vi "Dashboard Main.vi"() -> ()   [LabVIEW 2018]
uses:
  <vilib>/Utility/miscctls.llb/LVRowAndColumnTypeDef.ctl
  <vilib>/event_ctls.llb/eventvkey.ctl
  <vilib>/Rock Robotics/Network Tables/NT Read Numeric Array.vi
  <vilib>/Rock Robotics/Network Tables/NT Write Boolean.vi
  <vilib>/Rock Robotics/Network Tables/NT Read Boolean.vi
  <vilib>/Rock Robotics/WPI/Dashboard/WPI_DashboardLogging Global.vi
panel:
  in  "Camera Settings Right":T1={"Frame Rate"=30, "Compression"=30, "Size"=1, "DB Camera Config"=FALSE} {"Frame Rate" scale=1.0..30.0; "Compression" scale=100.0..-1.0; "Size" items=["640x480", "320x240", "160x120"]}
  in  "Camera Name Right":string(combo)="No Camera Selection"
  out "Camera Perf":string
  in  "Camera Settings":T1={"Frame Rate"=30, "Compression"=30, "Size"=1, "DB Camera Config"=FALSE} {"Frame Rate" scale=1.0..30.0; "Compression" scale=100.0..-1.0; "Size" items=["640x480", "320x240", "160x120"]}
  in  "TCP":refnum<k5>
  in  "Rec Mode":enum32{"Stop", "Record", "Playback"}(radio)
  out "Robot IP":string
  out "Image Message":string="Timeout in Camera Communications"
  in  "Dashboard Tab":T2(tab)
  in  "Bypass":bool
  out "Actif?":bool
  out "Limit Droite":bool
  out "Limit Gauche":bool
  out "Position Pendule":dbl
  out "Arr D":bool
  out "Arr G":bool
  out "Av D":bool
  out "Photocells":bool
  in  "Select Auto":string(combo)="Select Autonomous ..."
  out "NT Connection":bool
  out "MotorChart R":cluster{"Numeric":dbl, "Numeric":dbl}(graph)
  out "MotorChart L":cluster{"Numeric":dbl, "Numeric":dbl}(graph)
  out "MotorSliders R":cluster{"MotorSlide1":dbl, "MotorSlide2":dbl} {"MotorSlide2" scale=-1.0..1.0 scale format="%#_2e"; "MotorSlide1" scale=-1.0..1.0 scale format="%#_2e"}
  out "MotorSliders L":cluster{"MotorSlide1":dbl, "MotorSlide2":dbl} {"MotorSlide2" scale=-1.0..1.0 scale format="%#_2e"; "MotorSlide1" scale=-1.0..1.0 scale format="%#_2e"}
  out "Gyro":dbl(knob) scale=0.0..360.0
  out "JS1 Z":dbl(slide) scale=-1.0..1.0 scale format="%#_2e"
  out "JS1 Graph":cluster{"X":dbl, "Y":dbl}[](graph)
  out "JS1 Buttons":T3
  out "JS2 Z":dbl(slide) scale=-1.0..1.0 scale format="%#_2e"
  out "JS2 Graph":cluster{"X":dbl, "Y":dbl}[](graph)
  out "JS2 Buttons":T3
  out "Mode":T4(ring)=enum."Auto Disabled"
  out "Right Camera Perf":cluster{"Bandwidth (Mbps)":dbl, "FPS":dbl}
  out "Camera Image Right":T5(plugin-control)
  in  "DB/String 9":string
  in  "DB/String 8":string
  in  "DB/String 7":string
  in  "DB/String 6":string
  in  "DB/String 5":string
  in  "DB/String 4":string
  in  "DB/String 3":string
  in  "DB/String 2":string
  in  "DB/String 1":string
  in  "DB/String 0":string
  in  "DB/Slider 0":dbl(slide) scale=0.0..5.0
  in  "DB/Slider 1":dbl(slide) scale=0.0..5.0
  in  "DB/Slider 2":dbl(slide) scale=0.0..5.0
  in  "DB/Slider 3":dbl(slide) scale=0.0..5.0
  out "DB/LED 3":bool
  out "DB/LED 2":bool
  out "DB/LED 1":bool
  out "DB/LED 0":bool
  in  "DB/Button 3":bool
  in  "DB/Button 2":bool
  in  "DB/Button 1":bool
  in  "DB/Button 0":bool caption="New Name"
  in  "Test Slider":dbl(slide) scale=0.0..100.0 scale format="%#_3g"
  in  "On/Off":bool caption="Solenoid"
  in  "Test Name":u16(ring) items=["Select the test to run..."]
  in  "Test Tree":string(tree)
  in  "Motor":cluster{"Value":dbl, "Enable":bool} {"Value" scale=-1.0..1.0 scale format="%#_3g"}
  out "Progress":T6 {"Test Progress" scale=0.0..100.0}
  in  "Rev/Fwd":cluster{"Forward":bool, "Reverse":bool}
  in  "Test Ring":u16(ring) items=["Monochrome", "Color"]
  out "Cmd Status":string
  in  "Execute Command":bool
  in  "Command Params":string[][](table)
  in  "Command Selection":i32(listbox)
  in  "CheckList":i32(listbox)
  out "Tree":string(tree)
  out "Camera Image":T5(plugin-control)
  out "Background":bool
  in  "Camera Name":string(combo)="No Camera Selection"
  # "HW"
  # "HW"
  # "Joysticks"
  # "Drive Motors"
  # "Front"
  # "Right"
  # "Left"
  # "Back"
  # "This tab is a great place for autonomous settings and robot-specific values.\nPlace controls and indicators inside this tab and match name to\nDashboard Variables on robot. You can also delete this comment."
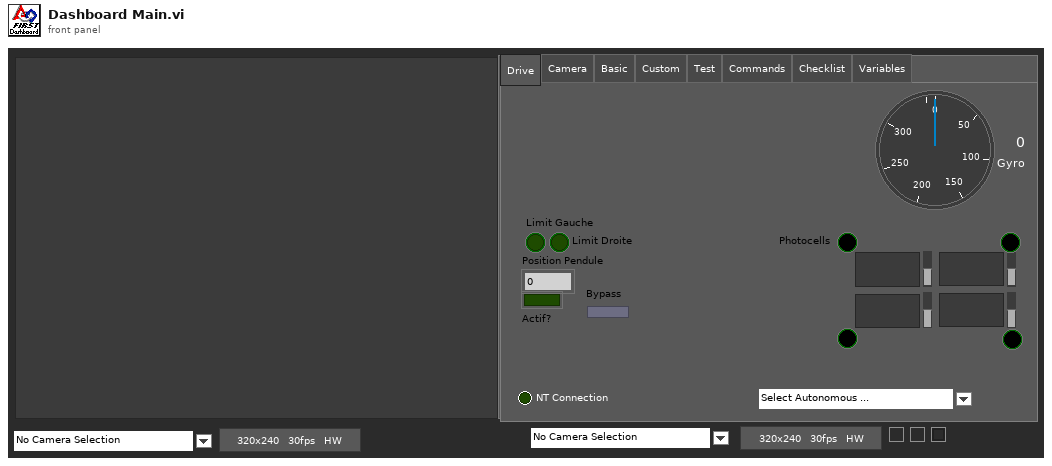
[diagram p1: front panel]
types:
  T1 = cluster{"Frame Rate":i32, "Compression":i32, "Size":u16, "DB Camera Config":bool}
  T2 = enum32{"Drive", "Camera", "Basic", "Custom", "Test", "Commands", "Checklist", "Variables"}
  T3 = cluster{bool, bool, bool, bool, bool, bool, bool, bool, bool, bool, bool, bool}
  T4 = enum8{"Tele-Op Disabled", "Tele-Op Enabled", "Auto Disabled", "Auto Enabled", "Test Disabled", "Test Enabled", "Disconnected", "No Code", "E-Stop"}
  T5 = typedef "IMAQ Image.ctl" = refnum<image>
  T6 = cluster{"Test Progress":u8, "Test Progress Text":string}
  T7 = cluster{"Save Path":path, "Interval (s)":dbl, "Keep":i32}
  T8 = typedef "Image Type" = u32
  T9 = cluster{"IDs":cluster{"RPC field ID":u16, "Unique ID":u16}, "String":string}
  T10 = cluster{"Error Strings":string, "Disable Counts":cluster{u16, u16}, "Rail Faults":cluster{u16, u16, u16}, "Robot IP":string, "DB Mode":u8, "Event Info":cluster{"Name":string, "Type":u8, "Number":u16, "Replay":u8}}
  T11 = cluster{"Storage":cluster{"Disk Free":u64, "RAM Block":u32, "RAM free":u32}, "CPU Utilization":cluster{"CPU % ISR":sgl, "CPU % Time Crit":sgl, "CPU % Timed Str":sgl, "CPU % High":sgl, "CPU % Above":sgl, "CPU % Normal":sgl, "CPU % Low":sgl}, "CAN":cluster{"% Bus Utilization":sgl, "Bus Off Cnt":u32, "TX_FIFO Full Cnt":u32, "Receive Error Cnt":u8, "Transmit Error Cnt":u8}, "HID":cluster{"HID Outputs":u32, "Rumble Low":u16, "Rumble High":u16}[]}
  T12 = cluster{"Status bits":cluster{"Test Mode":bool, "Autonomous":bool, "Enabled":bool, "Code Start":bool, "Brownout":bool, "Reserved 2":bool, "Reserved 3":bool, "E-Stop":bool}, "Code Trace":cluster{"Disabled":bool, "TeleOp":bool, "Auto":bool, "Test":bool}, "Controller Type":enum16{"unknown", "cRIO", "roboRio"}, "Code?":enum16{"unknown", "noCode", "code"}, "Battery V":dbl}
  T13 = cluster{"Control Bits":cluster{"TestMode":bool, "Autonomous":bool, "Enabled":bool, "FMS Present":bool, bool, bool, bool, "E-Stop":bool}, "Team Station ":u8, "Countdown":sgl, "Joystick Values":cluster{"Axes":dbl[], "Buttons":bool[], "POVs":i16[]}[]}
  T14 = cluster{"Axes":dbl[], "Buttons":bool[], "POVs":i16[]}[]
  T15 = cluster{"Axes":dbl[], "Buttons":bool[], "POVs":i16[]}
  T16 = cluster{"Buttons[0]":bool, "Buttons[1]":bool, "Buttons[2]":bool, "Buttons[3]":bool, "Buttons[4]":bool, "Buttons[5]":bool, "Buttons[6]":bool, "Buttons[7]":bool, "Buttons[8]":bool, "Buttons[9]":bool, "Buttons[10]":bool, "Buttons[11]":bool}
  T17 = cluster{"Camera Image":refnum<vi>, "Dashboard Tab":refnum<vi>, "Background":refnum<vi>, "Rec Mode":refnum<vi>, "Test Slider":refnum<vi>, "On/Off ":refnum<vi>, "Test Ring":refnum<vi>, "Rev/Fwd":refnum<vi>, "Test Name":refnum<vi>, "Motor":refnum<vi>, "Progress":refnum<vi>, "CheckList":refnum<vi>, "Tree":refnum<vi>, "Test Tree":refnum<vi>, "Command Params":refnum<vi>, "Command Selection":refnum<vi>, "Execute Command":refnum<vi>, "Cmd Status":refnum<vi>, "Camera Settings":refnum<vi>, "Camera Name":refnum<vi>, "Camera Perf":refnum<vi>, "Camera Settings Right":refnum<vi>, "Camera Name Right":refnum<vi>, "Camera Image Right":refnum<vi>}
  T18 = cluster{"Global Rectangle":i32[], "Contours":cluster{"Contour Type":u32, "ROI Type":u32, "Points":i32[]}[]}
  T19 = cluster{"Camera Name":string, string, "Saved DB Images Info":cluster{"Save Path":path, "Interval (s)":dbl, "Keep":i32}}
  T20 = cluster{"Camera Name Right":string, string, "Saved DB Images Info":cluster{"Save Path":path, "Interval (s)":dbl, "Keep":i32}}
  T21 = cluster{"Operation":enum16{"Update", "Clear"}, "Color Box":u32}[]
  T22 = typedef "eventvkey.ctl" = enum16{"ASCII", "Enter", "Return", "Shift", "Ctrl", "Alt", "Cmd", "Opt", "Caps", "NumLock", "Clear", "Break", "Up", "Down", "Left", "Right", "Insert", "Delete", "Home", "End", "PageUp", "PageDown", "Escape", "Help", "Pause", "ScrollLock", "F1", "F2", "F3", "F4", "F5", "F6", "F7", "F8", "F9", "F10", "F11", "F12", "F13", "F14", "F15", "F16", "F17", "F18", "F19", "F20", "F21", "F22", "F23", "F24", "Play", "VolumeUp", "VolumeDown", "Mute", "Two Byte Char"}
  T23 = cluster{"Image Size":bool, "Image Type":bool, "Pixel Value":bool, "ROI Information":bool, "Zoom Factor":bool}
  T24 = cluster{"Operation":enum16{"Update", "Clear"}, "Color Box":u32}
  T25 = typedef "LVRowAndColumnTypeDef.ctl" = cluster{"Row":i32, "Column":i32}
  T26 = cluster{"Shift":bool, "Ctrl":bool, "Alt":bool, "Cmd":bool, "Opt":bool}
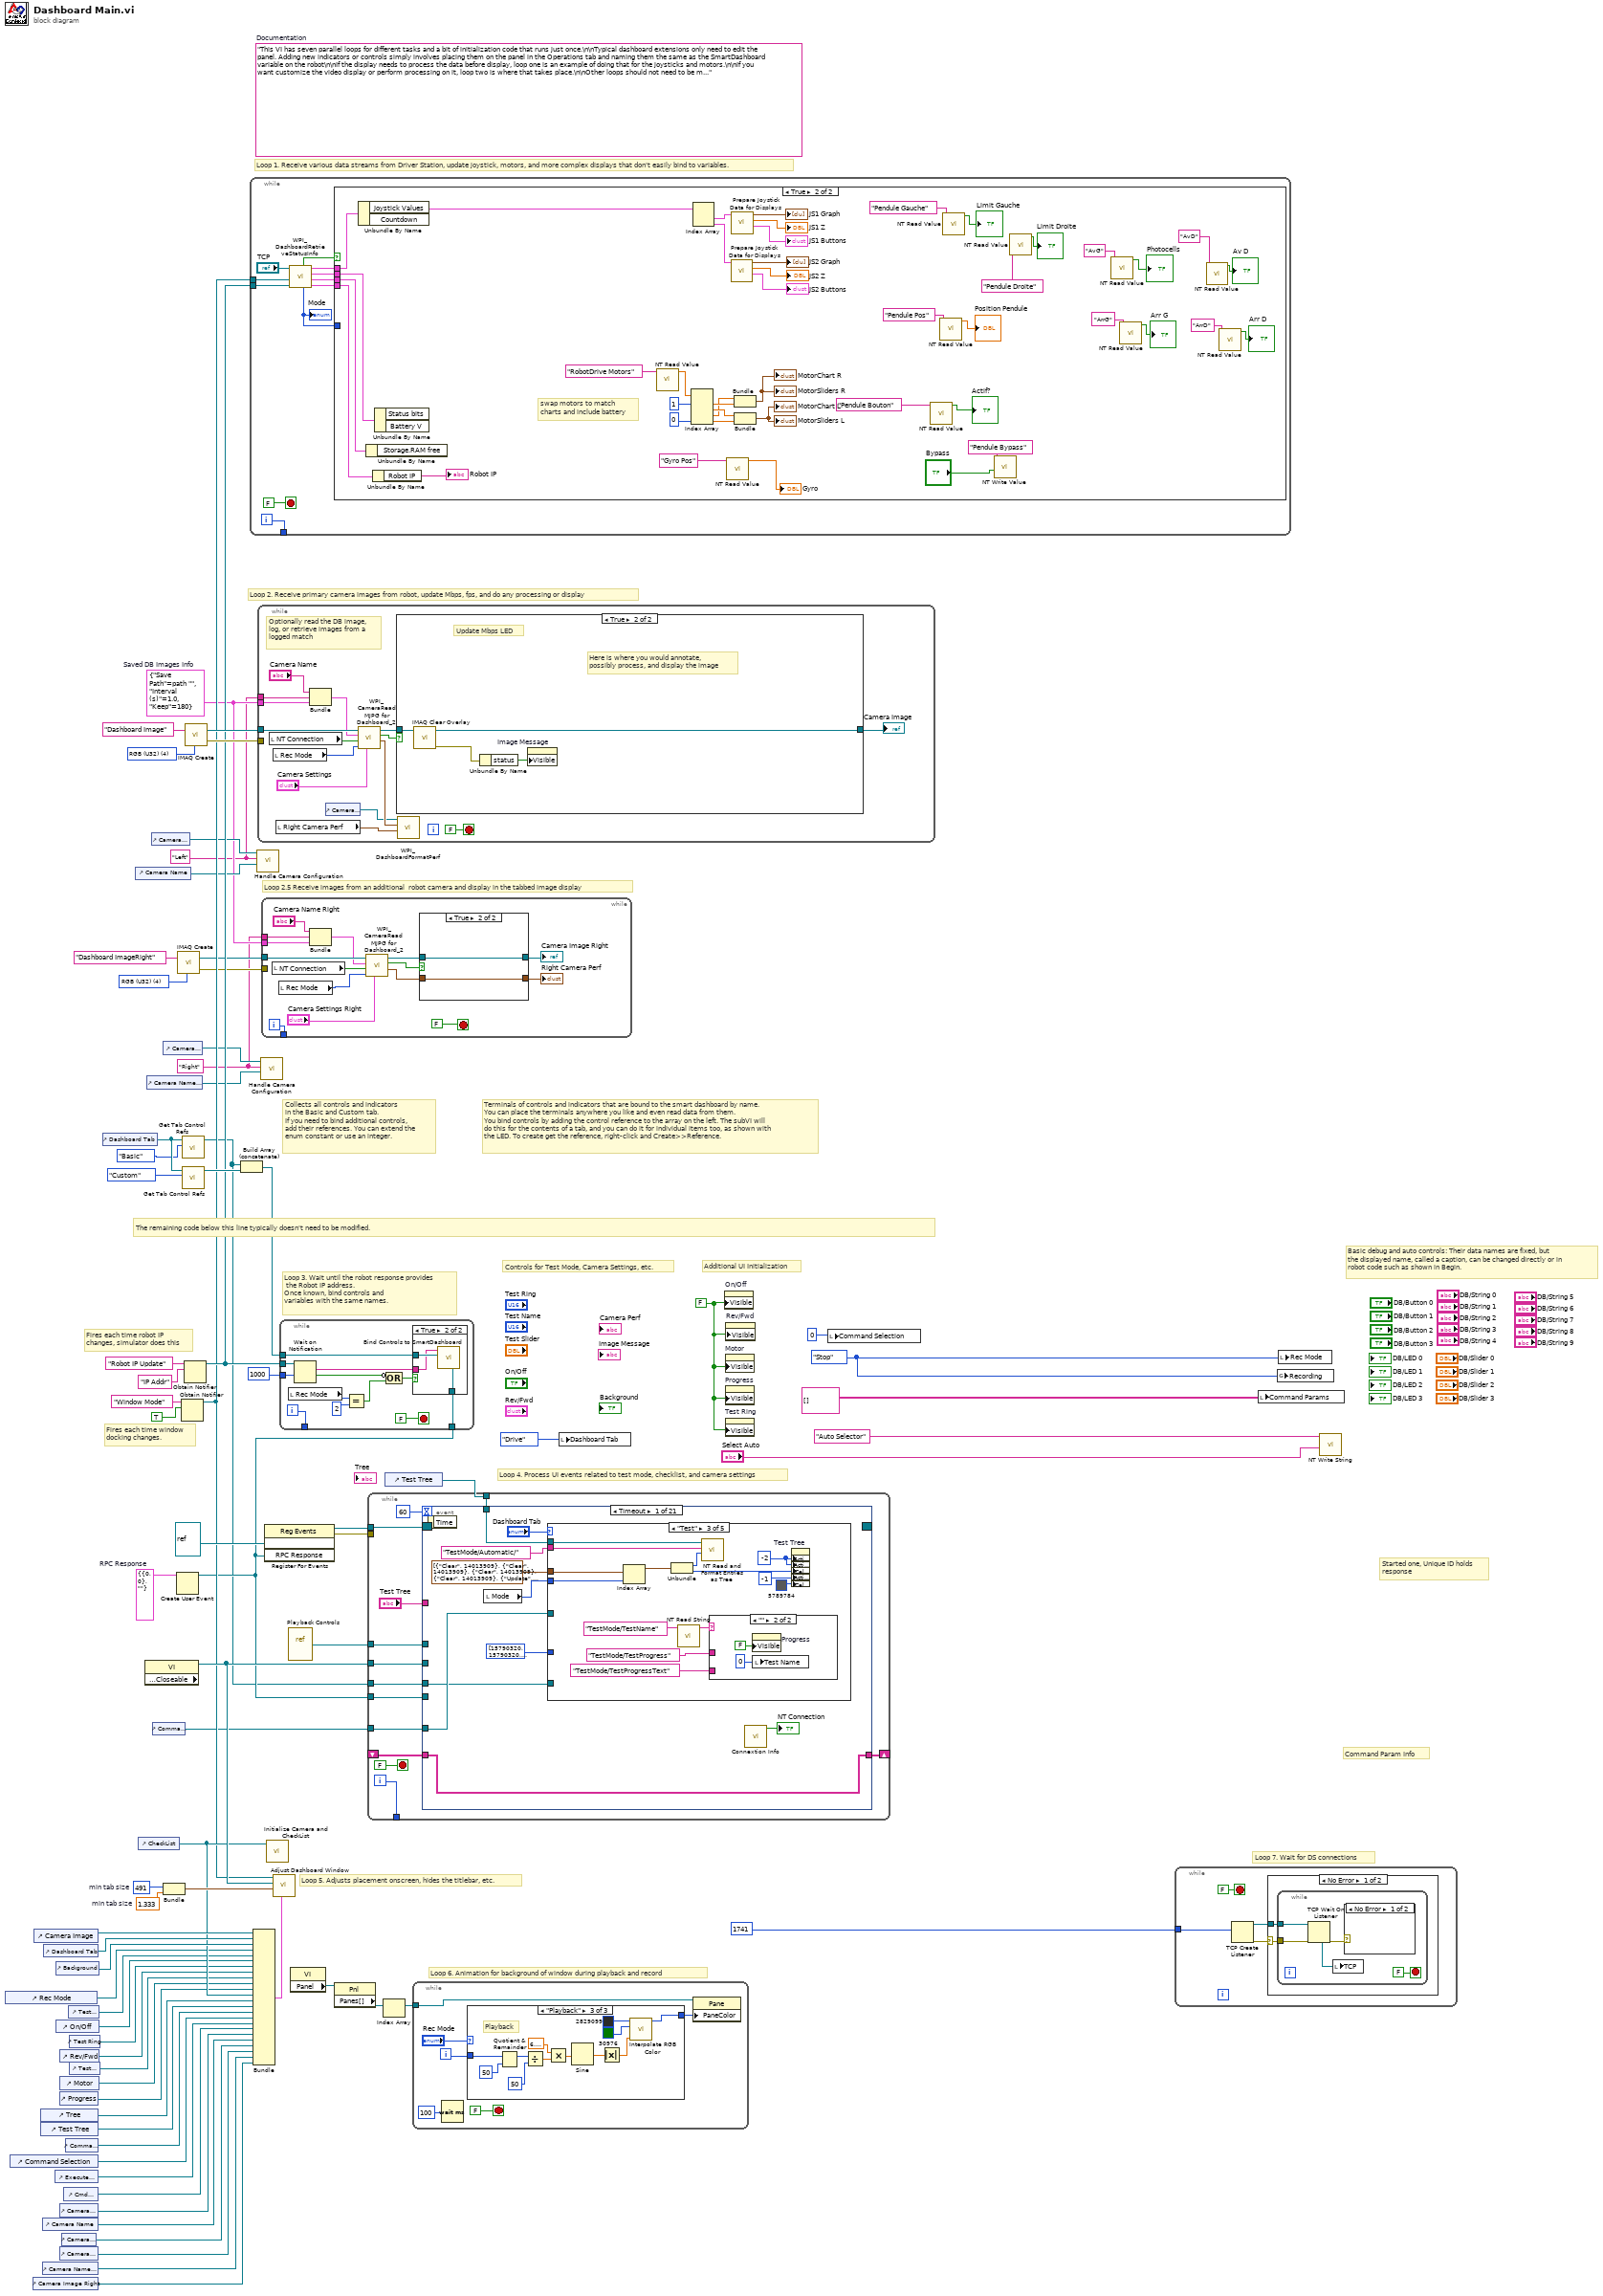
[diagram p0: block diagram]
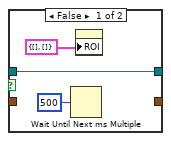
[diagram p2: hidden frame]
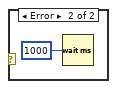
[diagram p3: hidden frame]
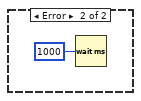
[diagram p4: hidden frame]
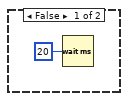
[diagram p5: hidden frame]
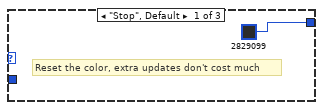
[diagram p6: hidden frame]
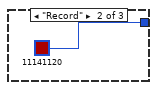
[diagram p7: hidden frame]
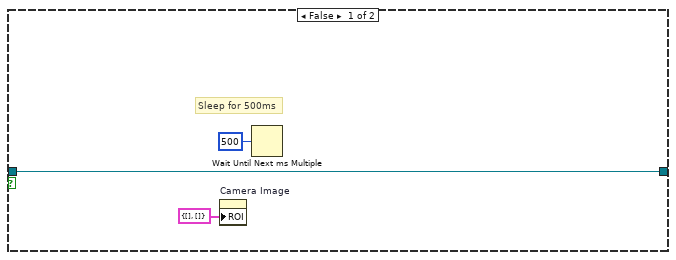
[diagram p9: hidden frame]
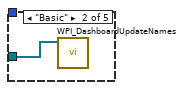
[diagram p11: hidden frame]
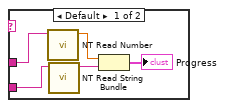
[diagram p12: hidden frame]
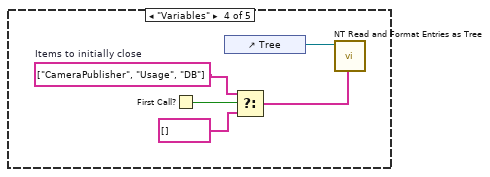
[diagram p13: hidden frame]
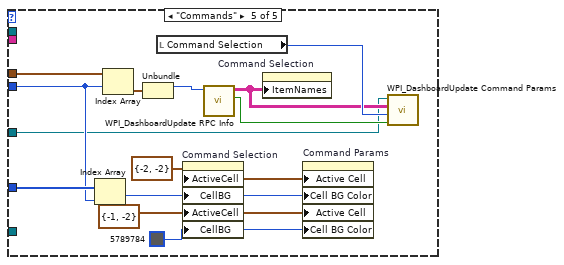
[diagram p14: hidden frame]
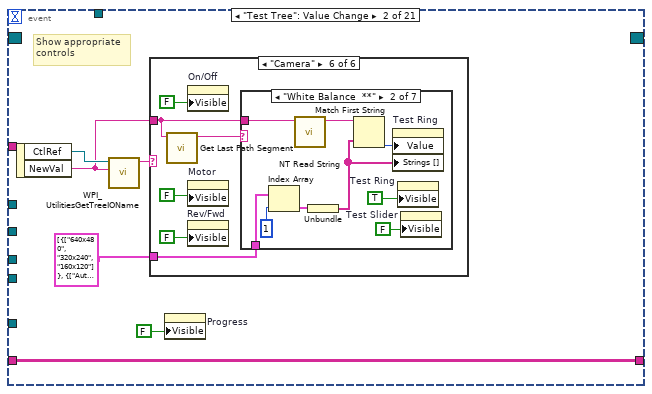
[diagram p15: hidden frame]
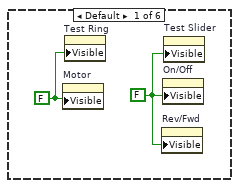
[diagram p16: hidden frame]
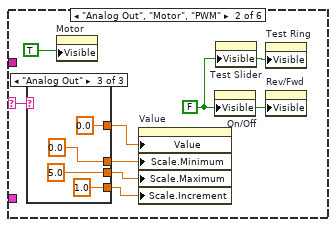
[diagram p17: hidden frame]
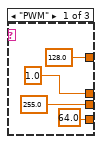
[diagram p18: hidden frame]
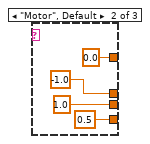
[diagram p19: hidden frame]
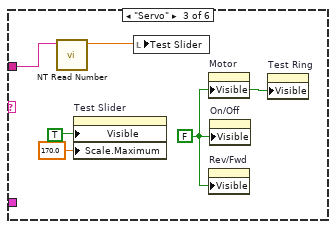
[diagram p20: hidden frame]
diagram:
  w3 = T7 {"Save Path"=path "", "Interval (s)"=1.0, "Keep"=180}  # Saved DB Images Info
  w2 = "Right"
  w1 = "Left"
  w13 = T8 4 items=["Grayscale (U8)", "Grayscale (I16)", "Grayscale (SGL)", "Complex (CSG)", "RGB (U32)", "HSL (U32)", "RGB (U64)"] ("Image Type")
  w29 = T9 {"IDs"={"RPC field ID"=0, "Unique ID"=0}, "String"=""}  # RPC Response
  w52 = 491  # min tab size
  w51 = 1.333  # min tab size
  w59 = enum32{"Stop", "Record", "Playback"}."Stop" ("Rec Mode")
  w36 = FALSE ("Visible")
  (unwired) "This VI has seven parallel loops for different tasks and a bit of initialization code that runs just once.\n\nTypical dashboard extensions only need to edit the panel. Adding new indicators or controls simply involves placing them on the panel in the Operations tab and naming them the same as the SmartDashboard variable on the robot\n\nIf the display needs to process the data before display, loop one is an example of doing that for the joysticks and motors.\n\nIf you want customize the video display or perform processing on it, loop two is where that takes place.\n\nOther loops should not need to be modified. They are pretty standard, and document the task they perform."  # Documentation
  w76 = T8 4 items=["Grayscale (U8)", "Grayscale (I16)", "Grayscale (SGL)", "Complex (CSG)", "RGB (U32)", "HSL (U32)", "RGB (U64)"] ("Image Type")
  # "Loop 2.5 Receive images from an additional  robot camera and display in the tabbed image display"
  # "Command Param Info"
  # "Started one, Unique ID holds\nresponse"
  # "Loop 7. Wait for DS connections"
  # "Basic debug and auto controls: Their data names are fixed, but\nthe displayed name, called a caption, can be changed directly or in\nrobot code such as shown in Begin."
  # "Controls for Test Mode, Camera Settings, etc."
  # "Additional UI Initialization"
  # "Loop 6. Animation for background of window during playback and record"
  # "Fires each time robot IP\nchanges, simulator does this"
  # "Fires each time window\ndocking changes."
  # "Collects all controls and indicators\nin the Basic and Custom tab.\nIf you need to bind additional controls,\nadd their references. You can extend the\nenum constant or use an integer."
  # "The remaining code below this line typically doesn't need to be modified."
  # "Loop 4. Process UI events related to test mode, checklist, and camera settings"
  # "Terminals of controls and indicators that are bound to the smart dashboard by name.\nYou can place the terminals anywhere you like and even read data from them.\nYou bind controls by adding the control reference to the array on the left. The subVI will\ndo this for the contents of a tab, and you can do it for individual items too, as shown with\nthe LED. To create get the reference, right-click and Create>>Reference."
  # "Loop 3. Wait until the robot response provides\n the Robot IP address.\nOnce known, bind controls and\nvariables with the same names."
  # "Loop 5. Adjusts placement onscreen, hides the titlebar, etc."
  # "Loop 1. Receive various data streams from Driver Station, update joystick, motors, and more complex displays that don't easily bind to variables."
  # "Loop 2. Receive primary camera images from robot, update Mbps, fps, and do any processing or display"
  n1 = control-ref of="Rec Mode"() -> (w42:refnum<vi>)
  n2 = control-ref of="Command Selection"() -> (w28:refnum<vi>)
  n3 = control-ref of="Camera Image Right"() -> (w6:refnum<vi>)
  n4 = control-ref of="Camera Image"() -> (w54:refnum<vi>)
  n5 = control-ref of="Tree"() -> (w46:refnum<vi>)
  n6 = control-ref of="Test Tree"() -> (w45:refnum<vi>)
  n7 = control-ref of="Camera Name"() -> (w19:refnum<vi>)
  n8 = control-ref of="Camera Name Right"() -> (w7:refnum<vi>)
  n9 = control-ref of="Dashboard Tab"() -> (w53:refnum<vi>)
  n10 = control-ref of="Execute Command"() -> (w30:refnum<vi>)
  n11 = control-ref of="Background"() -> (w49:refnum<vi>)
  n12 = control-ref of="On/Off"() -> (w40:refnum<vi>)
  n13 = control-ref of="Progress"() -> (w37:refnum<vi>)
  n14 = control-ref of="Camera Settings"() -> (w20:refnum<vi>)
  n15 = control-ref of="Camera Settings Right"() -> (w8:refnum<vi>)
  n16 = control-ref of="Rev/Fwd"() -> (w38:refnum<vi>)
  n17 = control-ref of="Motor"() -> (w43:refnum<vi>)
  n18 = control-ref of="Camera Perf"() -> (w18:refnum<vi>)
  n19 = control-ref of="Cmd Status"() -> (w24:refnum<vi>)
  n20 = control-ref of="Command Params"() -> (w31:refnum<vi>)
  n21 = control-ref of="Test Slider"() -> (w41:refnum<vi>)
  n22 = control-ref of="Test Ring"() -> (w39:refnum<vi>)
  n23 = control-ref of="Test Name"() -> (w44:refnum<vi>)
  n24 = control-ref of="Dashboard Tab"() -> (w57:refnum<vi>)
  n25 = control-ref of="Camera Name"() -> (w21:refnum<vi>)
  n26 = control-ref of="CheckList"() -> (w47:refnum<vi>)
  n27 = property class="VI" props=["Front Panel.Closeable"]() -> (reference out=w58:refnum<vi>)  [unwired: 2 in, 2 out]
  n28 = control-ref of="Camera Name Right"() -> (w9:refnum<vi>)
  n29 = control-ref of="Camera Settings"() -> (w22:refnum<vi>)
  n30 = control-ref of="Command Params"() -> (w23:refnum<vi>)
  n31 = control-ref of="Camera Settings Right"() -> (w10:refnum<vi>)
  n32 = Bundle("min tab size"=w52, "min tab size"=w51) -> (w50:cluster{"min tab size":i32, "min tab size":dbl})  [unwired: 1 in]
  n33 = Create User Event(user event datatype=w29) -> (user event=w25:refnum<user-event>)  [unwired: 1 in, 1 out]
  n34 = call "IMAQ Create"("Image Name"="Dashboard ImageRight", "Image Type"=w13) -> ("New Image"=w12:T5, "error out"=w11:errorcluster)  [unwired: 2 in, 1 out]
  n35 = Obtain Notifier(name (unnamed)="Window Mode", notification data type=TRUE) -> (notifier out=w34:refnum<notifier>)  [unwired: 2 in, 2 out]
  n36 = call <vilib>:"Get Tab Control Refs.vi"("Page Index"=T2."Basic" ("Dashboard Tab"), "TabControl in"=w57) -> ("ControlsOnPage"=w17:refnum<vi>[])  [unwired: 9 in]
  n37 = call <vilib>:"Get Tab Control Refs.vi"("Page Index"=T2."Custom" ("Dashboard Tab"), "TabControl in"=w57) -> ("ControlsOnPage"=w56:refnum<vi>[])  [unwired: 9 in]
  n38 = Obtain Notifier(name (unnamed)="Robot IP Update", notification data type="IP Addr" ("name (unnamed)")) -> (notifier out=w35:refnum<notifier>)  [unwired: 2 in, 2 out]
  n39 = call "IMAQ Create"("Image Name"="Dashboard Image", "Image Type"=w76) -> ("New Image"=w74:T5, "error out"=w73:errorcluster)  [unwired: 2 in, 1 out]
  n40 = Build Array (concatenate)(w17, w56) -> (w55:refnum<vi>[])
  n41 = while {
    tunnel: [w86] -> _
    tunnel: w35 -> [w80]
    tunnel: w34 -> [w77]
    i -> [w86]
    stop <- FALSE stop-if-true
    n42 = call <vilib>:"WPI_DashboardRetrieveStatusInfo.vi"("Binding Refnum"=w80, "Window Mode Notifier"=w77, "TCP Cnx"="TCP") -> ("Power and Errors"=w81:T10, "Robot Metrics"=w84:T11, "Status Info"=w85:T12, "Control Info"=w82:T13, "Robot Mode"=w79:T4, "Process?"=w83:bool)  [unwired: 3 in]
    "Mode" <- w79
    n43 = case shown="True" w83 {
      tunnel: w85 -> [_ w132]
      tunnel: w84 -> [_ w131]
      tunnel: w82 -> [_ w130]
      tunnel: w81 -> [_ w129]
      tunnel: w79 -> [_ _]
      frame False {
        n44 = Wait (ms)(milliseconds to wait=u32 20) -> ()  [unwired: 1 out]
      }
      frame True {
        # "swap motors to match\ncharts and include battery"
        n45 = Unbundle By Name(w130) -> ("Joystick Values"=w120:T14)  [unwired: 1 out]
        n46 = Unbundle By Name(w131) -> ()  [unwired: 1 out]
        n47 = Unbundle By Name(w129) -> ("Robot IP"=→"Robot IP":string)
        n48 = Unbundle By Name(w132) -> ()  [unwired: 2 out]
        n49 = call-poly <vilib>:"NT Read Value.vi"("Name"="RobotDrive Motors") -> ("Numeric Array"=w110:dbl[])  [unwired: 9 in, 1 out]
        n50 = Index Array(array=w110, index #1=1, index #4=0) -> (element #1=w124:dbl, element #2=w125:dbl, element #3=w123:dbl, element #4=w128:dbl)  [unwired: 2 in]
        n51 = Index Array(array=w120) -> (element #1=w119:T15, element #2=w115:T15)  [unwired: 2 in]
        n52 = call-poly <vilib>:"NT Read Value.vi"("Name"="Gyro Pos") -> ("Numeric"=→"Gyro":dbl)  [unwired: 9 in, 1 out]
        n53 = call "Prepare Joystick Data for Displays.vi"("Joystick Values"=w115) -> ("Buttons"=→"JS2 Buttons":T16, "Z Axis"=→"JS2 Z":dbl, "Cartesian Data"=→"JS2 Graph":cluster{"X axis":dbl, "X axis":dbl}[])  [unwired: 8 in]
        n54 = call "Prepare Joystick Data for Displays.vi"("Joystick Values"=w119) -> ("Buttons"=→"JS1 Buttons":T16, "Z Axis"=→"JS1 Z":dbl, "Cartesian Data"=→"JS1 Graph":cluster{"X axis":dbl, "X axis":dbl}[])  [unwired: 8 in]
        n55 = Bundle("Numeric"=w123, "Numeric"=w124) -> (→"MotorChart R" →"MotorSliders R":cluster{"Numeric":dbl, "Numeric":dbl})  [unwired: 1 in]
        n56 = Bundle("Numeric"=w125, "Numeric"=w128) -> (→"MotorChart L" →"MotorSliders L":cluster{"Numeric":dbl, "Numeric":dbl})  [unwired: 1 in]
        n57 = call-poly <vilib>:"NT Read Value.vi"("Name"="Pendule Bouton") -> ("Boolean"=→"Actif?":bool)  [unwired: 9 in, 1 out]
        n58 = call-poly <vilib>:"NT Read Value.vi"("Name"="Pendule Pos") -> ("Numeric"=→"Position Pendule":dbl)  [unwired: 9 in, 1 out]
        n59 = call-poly <vilib>:"NT Read Value.vi"("Name"="Pendule Gauche") -> ("Boolean"=→"Limit Gauche":bool)  [unwired: 9 in, 1 out]
        n60 = call-poly <vilib>:"NT Write Value.vi"("Boolean"="Bypass", "Name"="Pendule Bypass") -> ()  [unwired: 9 in, 1 out]
        n61 = call-poly <vilib>:"NT Read Value.vi"("Name"="Pendule Droite") -> ("Boolean"=→"Limit Droite":bool)  [unwired: 9 in, 1 out]
        n62 = call-poly <vilib>:"NT Read Value.vi"("Name"="AvG") -> ("Boolean"=→"Photocells":bool)  [unwired: 9 in, 1 out]
        n63 = call-poly <vilib>:"NT Read Value.vi"("Name"="ArrG") -> ("Boolean"=→"Arr G":bool)  [unwired: 9 in, 1 out]
        n64 = call-poly <vilib>:"NT Read Value.vi"("Name"="AvD") -> ("Boolean"=→"Av D":bool)  [unwired: 9 in, 1 out]
        n65 = call-poly <vilib>:"NT Read Value.vi"("Name"="ArrD") -> ("Boolean"=→"Arr D":bool)  [unwired: 9 in, 1 out]
      }
    }
  }
  n66 = Bundle("Camera Image"=w54, "Dashboard Tab"=w53, "Background"=w49, "Rec Mode"=w42, "Test Slider"=w41, "On/Off"=w40, "Test Ring"=w39, "Rev/Fwd"=w38, "Test Name"=w44, "Motor"=w43, "Progress"=w37, "CheckList"=w47, "Tree"=w46, "Test Tree"=w45, "Command Params"=w31, "Command Selection"=w28, "Execute Command"=w30, "Cmd Status"=w24, "Camera Settings"=w20, "Camera Name"=w19, "Camera Perf"=w18, "Camera Settings Right"=w8, "Camera Name Right"=w7, "Camera Image Right"=w6) -> (w48:T17)  [unwired: 1 in]
  n67 = call "Handle Camera Configuration.vi"("CameraNameRef"=w21, "Display Name"=w1, "ClusterRef"=w22) -> ()  [unwired: 9 in]
  n68 = while {
    tunnel: w74 -> [w146]
    tunnel: w73 -> [_]
    tunnel: w3 -> [w139]
    tunnel: w1 -> [w136]
    stop <- FALSE stop-if-true
    # "Optionally read the DB image,\nlog, or retrieve images from a\nlogged match"
    n69 = local read "NT Connection"() -> (w140:bool)
    n70 = local read "Rec Mode"() -> (w143:enum32{"Stop", "Record", "Playback"})
    n71 = local read "Right Camera Perf"() -> (w134:cluster{"Bandwidth (Mbps)":dbl, "FPS":dbl})
    n72 = Bundle("Camera Name"="Camera Name", w136, "Saved DB Images Info"=w139) -> (w138:T19)  [unwired: 1 in]
    n73 = control-ref of="Camera Perf"() -> (w133:refnum<vi>)
    n74 = call <vilib>:"WPI_CameraRead MJPG for Dashboard_2.vi"("Camera Settings"="Camera Settings", "Rec Mode"=w143, "NT Connection"=w140, "Capture Info"=w138, "Image in"=w146) -> ("perf info"=w135:cluster{"Bandwidth (Mbps)":dbl, "fps":dbl}, "Active"=w144:bool, "Image\\ out"=w145:T5)  [unwired: 4 in]
    n75 = case shown="True" w144 {
      tunnel: w145 -> [w149 w152]
      tunnel: [w149 w151] -> w141
      frame False {
        # "Sleep for 500ms"
        n76 = property on="Camera Image" class="ImageControl"("ROI"=T18 {"Global Rectangle"=[], "Contours"=[]}) -> ()  [unwired: 2 in, 2 out]
        n77 = Wait Until Next ms Multiple(millisecond multiple=u32 500) -> ()  [unwired: 1 out]
      }
      frame True {
        # "Here is where you would annotate,\npossibly process, and display the image"
        # "Update Mbps LED"
        n78 = call "IMAQ Clear Overlay"("Image"=w152) -> ("error out"=w153:errorcluster, "Image Out"=w151:T5)  [unwired: 2 in, 7 out]
        n79 = Unbundle By Name(w153) -> ("status"=w154:bool)
        n80 = property on="Image Message" class="Str"("Visible"=w154) -> ()  [unwired: 2 in, 2 out]
      }
    }
    "Camera Image" <- w141
    n81 = call <vilib>:"WPI_DashboardFormatPerf.vi"("Right Camera Perf"=w134, "Performance"=w135, "String in"=w133) -> ()  [unwired: 9 in]
  }
  n82 = call "Handle Camera Configuration.vi"("CameraNameRef"=w9, "Display Name"=w2, "ClusterRef"=w10) -> ()  [unwired: 9 in]
  n83 = while {
    tunnel: w12 -> [w169]
    tunnel: w11 -> [_]
    tunnel: [w164] -> _
    tunnel: w3 -> [w160]
    tunnel: w2 -> [w157]
    i -> [w164]
    stop <- FALSE stop-if-true
    n84 = local read "NT Connection"() -> (w161:bool)
    n85 = local read "Rec Mode"() -> (w168:enum32{"Stop", "Record", "Playback"})
    n86 = Bundle("Camera Name Right"="Camera Name Right", w157, "Saved DB Images Info"=w160) -> (w159:T20)  [unwired: 1 in]
    n87 = call <vilib>:"WPI_CameraRead MJPG for Dashboard_2.vi"("Camera Settings"="Camera Settings Right", "Rec Mode"=w168, "NT Connection"=w161, "Capture Info"=w159, "Image in"=w169) -> ("perf info"=w155:cluster{"Bandwidth (Mbps)":dbl, "fps":dbl}, "Active"=w163:bool, "Image\\ out"=w166:T5)  [unwired: 4 in]
    n88 = case shown="True" w163 {
      tunnel: w166 -> [w171 w174]
      tunnel: [w171 w174] -> w162
      tunnel: [_ w173] -> w156
      tunnel: w155 -> [_ w173]
      frame False {
        n89 = Wait Until Next ms Multiple(millisecond multiple=u32 500) -> ()  [unwired: 1 out]
        n90 = property on="Camera Image Right" class="ImageControl"("ROI"=T18 {"Global Rectangle"=[], "Contours"=[]}) -> ()  [unwired: 2 in, 2 out]
      }
      frame True {
      }
    }
    "Camera Image Right" <- w162
    "Right Camera Perf" <- w156
  }
  n91 = register-events(refnum<vi> refnum, w25) -> (reference out=w63:refnum<event-registration>, error out=w62:errorcluster)  [unwired: 2 in]
  n92 = call "Initialize Camera and CheckList.vi"("ListBox in"=w47) -> ()  [unwired: 11 in]
  n93 = call "Adjust Dashboard Window.vi"("Sizing Refnums"=w48, "Size Constraints"=w50, "VI"=w58, "WIn Mode"=w34) -> ()  [unwired: 8 in]
  n94 = while {
    tunnel: w55 -> [w186]
    tunnel: w35 -> [w184]
    tunnel: [w182] -> _
    tunnel: u32 1000 ("milliseconds to wait") -> [w181]
    tunnel: w25 -> [w175]
    i -> [w182]
    stop <- FALSE stop-if-true
    n95 = local read "Rec Mode"() -> (w177:enum32{"Stop", "Record", "Playback"})
    n96 = Wait on Notification(notifier=w184, timeout in ms (-1)=w181) -> (notification=w183:string, timed out?=w179:bool)  [unwired: 2 in, 2 out]
    n97 = Equal?(x=w177, y=u16 2 ("Rec Mode")) -> (x = y?=w178:bool)
    n98 = Compound Arithmetic op=OR(invert w179, w178) -> (w180:bool)
    n99 = case shown="True" w180 {
      tunnel: w186 -> [_ w189]
      tunnel: w183 -> [_ w188]
      tunnel: w175 -> [_ w187]
      frame False {
      }
      frame True {
        n100 = call <vilib>:"Bind Controls to SmartDashboard.vi"("RPC ref"=w187, "Bound Control Refs"=w189, "Server IP Address"=w188) -> ()  [unwired: 9 in]
      }
    }
  }
  n101 = vi-ref "Playback Controls.vi"() -> (w64:refnum<vi>)
  n102 = property class="VI"() -> ("Panel"=w66:refnum<vi>)  [unwired: 2 in, 2 out]
  n103 = property class="Pnl"(reference=w66) -> ("Panes[]"=w67:refnum<vi>[])  [unwired: 1 in, 2 out]
  n104 = Index Array(array=w67) -> (element=w65:refnum<vi>)  [unwired: 1 in]
  n105 = control-ref of="Test Tree"() -> (w68:refnum<vi>)
  n106 = while {
    tunnel: [w199] -> _
    tunnel: w68 -> [w198]
    tunnel: w64 -> [w197]
    tunnel: w63 -> [w196]
    tunnel: w62 -> [_]
    tunnel: w58 -> [w195]
    tunnel: w25 -> [w194]
    tunnel: w23 -> [w193]
    shift-right: [w192] -> _
    shift-left: _ -> [w191]
    tunnel: w17 -> [w190]
    i -> [w199]
    stop <- FALSE stop-if-true
    n107 = event shown="[0] Timeout" {
      selector: w196 -> [_ _ _ _ _ _ _ _ _ _ _ _ _ _ _ _ _ _ _ _ _]
      dyn-events: [_ _ _ _ _ _ _ _ _ _ _ _ _ _ _ _ w459 _ _ _ _] -> _
      timeout: u32 60 ("milliseconds to wait") -> [_ _ _ _ _ _ _ _ _ _ _ _ _ _ _ _ _ _ _ _ _]
      tunnel: w198 -> [w211 _ _ _ _ _ _ _ _ _ _ _ _ _ _ _ _ _ _ _ _]
      tunnel: "Test Tree" -> [_ _ _ _ _ _ _ _ _ _ _ w426 w434 w436 w440 w448 _ _ _ _ _]
      tunnel: w197 -> [_ _ _ _ _ _ _ _ _ _ _ _ _ _ _ _ w461 _ w479 _ _]
      tunnel: w195 -> [_ _ _ _ _ _ _ _ _ _ _ _ _ _ _ _ w457 _ _ _ _]
      tunnel: w194 -> [_ _ _ _ _ _ _ _ _ _ _ _ _ _ _ _ w455 _ _ _ _]
      tunnel: w193 -> [w206 _ _ _ _ _ w377 _ _ _ _ _ _ _ _ _ _ _ _ _ _]
      tunnel: [w205 w254 w356 w361 w370 w374 w375 w384 w394 w401 w413 w425 w432 w435 w439 w447 w454 w474 w476 w480 w493] -> w192
      tunnel: w191 -> [w205 w254 w356 w361 w370 w374 w375 _ _ w401 w413 w425 w432 w435 w439 w447 w454 w474 w476 w480 w493]
      tunnel: w190 -> [w203 _ _ _ _ _ _ _ _ _ _ _ _ _ _ _ _ _ _ _ _]
      event Timeout {
        n108 = event-data() -> ()  [unwired: 1 in, 1 out]
        n109 = local read "Mode"() -> (w208:T4)
        n110 = case shown="\"Test\"" "Dashboard Tab" {
          tunnel: w211 -> [_ _ w227 _ _]
          tunnel: "TestMode/Automatic/" ("Name Pattern") -> [_ _ w226 _ _]
          tunnel: T21 [{"Operation"=enum."Clear", "Color Box"=14013909}, {"Operation"=enum."Clear", "Color Box"=14013909}, {"Operation"=enum."Clear", "Color Box"=14013909}, {"Operation"=enum."Clear", "Color Box"=14013909}, {"Operation"=enum."Update", "Color Box"=14013909}, {"Operation"=enum."Update", "Color Box"=16777215}, {"Operation"=enum."Clear", "Color Box"=14013909}, {"Operation"=enum."Clear", "Color Box"=14013909}, {"Operation"=enum."Clear", "Color Box"=14013909}] -> [_ _ w219 _ w247]
          tunnel: w208 -> [_ _ w218 _ w246]
          tunnel: u32[] [15790320, 15790320, 15790320, 15790320, 16777215, 16777215, 15790320, 15790320, 15790320] -> [_ _ _ _ w252]
          tunnel: w206 -> [_ _ _ _ w240]
          tunnel: w203 -> [_ w213 _ _ _]
          frame "Custom", Default {
          }
          frame "Basic" {
            n111 = call <vilib>:"WPI_DashboardUpdateNames.vi"("Controls on Tab"=w213) -> ()  [unwired: 11 in]
          }
          frame "Test" {
            w225 = -2 ("Active Item:Row Number")
            n112 = Index Array(array=w219, index=w218) -> (element=w220:T24)
            n113 = Unbundle(w220) -> ("Operation"=w221:enum16{"Update", "Clear"}, "Color Box"=w222:u32)
            n114 = call <vilib>:"NT Read String.vi"("Name"="TestMode/TestName") -> ("String"=w216:string)  [unwired: 9 in, 1 out]
            n115 = call <vilib>:"NT Read and Format Entries as Tree.vi"("Operation"=w221, "Name Pattern"=w226, "Tree Refnum"=w227) -> ()  [unwired: 7 in, 2 out]
            n116 = case shown="\"\"" w216 {
              tunnel: "TestMode/TestProgress" ("Name") -> [w229 _]
              tunnel: "TestMode/TestProgressText" ("Name") -> [w228 _]
              frame Default {
                n117 = call <vilib>:"NT Read Number.vi"("Name"=w229) -> ("Numeric"=w230:dbl)  [unwired: 9 in, 1 out]
                n118 = call <vilib>:"NT Read String.vi"("Name"=w228) -> ("String"=w231:string)  [unwired: 9 in, 1 out]
                n119 = Bundle("Numeric"=w230, "String"=w231) -> (→"Progress":cluster{"Numeric":dbl, "String":string})  [unwired: 1 in]
              }
              frame "" {
                n120 = property on="Progress" class="Clust (strict)"("Visible"=FALSE) -> ()  [unwired: 2 in, 2 out]
                n121 = local write "Test Name"(u16 0) -> ()
              }
            }
            n122 = property on="Test Tree" class="Tree (strict)"("Active Item Row Number"=w225, "ActiveColNum"=w225, "CellBG"=w222, "Active Item Row Number"=-1 ("Active Item:Row Number"), "CellBG"=u32 5789784 ("Color Box")) -> ()  [unwired: 2 in, 2 out]
          }
          frame "Variables" {
            w237 = string[] ["CameraPublisher", "Usage", "DB"]  # Items to initially close
            n123 = First Call?() -> (First Call?: T/F=w238:bool)
            n124 = control-ref of="Tree"() -> (w239:refnum<vi>)
            n125 = Select(t=w237, s=w238, f=string[] []) -> (s? t:f=w235:string[])
            n126 = call <vilib>:"NT Read and Format Entries as Tree.vi"("Tags to  Close"=w235, "Tree Refnum"=w239) -> ()  [unwired: 8 in, 2 out]
          }
          frame "Commands" {
            w248 = u32 5789784 ("Color Box")
            w249 = T25 {"Row"=-1, "Column"=-2} ("Active Cell:Active Cell")
            w251 = T25 {"Row"=-2, "Column"=-2} ("Active Cell:Active Cell")
            n127 = Index Array(array=w252, index=w246) -> (element=w250:u32)
            n128 = Index Array(array=w247, index=w246) -> (element=w245:T24)
            n129 = Unbundle(w245) -> ("Operation"=w244:enum16{"Update", "Clear"})  [unwired: 1 out]
            n130 = local read "Command Selection"() -> (w243:i32)
            n131 = property on="Command Selection" class="MCListbox (strict)"("ActiveCell"=w251, "CellBG"=w250, "ActiveCell"=w249, "CellBG"=w248) -> ()  [unwired: 2 in, 2 out]
            n132 = call <vilib>:"WPI_DashboardUpdate RPC Info.vi"("Operation"=w244) -> ("update"=w242:bool, "commands"=w241:string[][])  [unwired: 9 in]
            n133 = property on="Command Selection" class="MCListbox (strict)"("ItemNames"=w241) -> ()  [unwired: 2 in, 2 out]
            n134 = property on="Command Params" class="Tbl (strict)"("Active Cell"=w251, "Cell BG Color"=w250, "Active Cell"=w249, "Cell BG Color"=w248) -> ()  [unwired: 2 in, 2 out]
            n135 = call <vilib>:"WPI_DashboardUpdate Command Params.vi"("Update"=w242, "NewVal"=w243, "Commands"=w241, "Param Tbl"=w240) -> ()  [unwired: 7 in, 1 out]
          }
        }
        n136 = call <vilib>:"Connextion Info.vi"() -> ("Connected"=→"NT Connection":bool)  [unwired: 10 in, 1 out]
      }
      event "Test Tree": Value Change {
        # "Show appropriate\ncontrols"
        n137 = event-data() -> ("CtlRef"=w257:refnum<vi>, "NewVal"=w255:string)  [unwired: 1 in]
        n138 = call <vilib>:"WPI_UtilitiesGetTreeIOName.vi"("NewVal"=w255, "TreeControl in"=w257) -> ("I/O Name"=w258:string)  [unwired: 9 in]
        n139 = case shown="\"Camera\"" w258 {
          selector: w258 -> [_ w265 _ w287 w296 _]
          tunnel: w255 -> [_ _ w284 w286 _ w303]
          tunnel: cluster{string[]}[] [{["640x480", "320x240", "160x120"]}, {["Auto", "Fixed indoor", "Fixed outdoor 1", "Fixed outdoor 2", "Fixed fluorescent 1", "Fixed fluorescent 2", "Hold current"]}, {["Auto", "Flicker-free 50 Hz", "Flicker-free 60 Hz", "Hold current"]}, {["None", "Prioritize frame rate", "Prioritize image quality"]}, {["Monochrome", "Color"]}] -> [_ _ _ _ _ w302]
          frame Default {
            w260 = FALSE ("Visible")
            w259 = FALSE ("Visible")
            n140 = property on="Motor" class="Clust (strict)"("Visible"=w259) -> ()  [unwired: 2 in, 2 out]
            n141 = property on="Test Ring" class="Ring (strict)"("Visible"=w259) -> ()  [unwired: 2 in, 2 out]
            n142 = property on="Rev/Fwd" class="Clust (strict)"("Visible"=w260) -> ()  [unwired: 2 in, 2 out]
            n143 = property on="On/Off" class="Bool (strict)"("Visible"=w260) -> ()  [unwired: 2 in, 2 out]
            n144 = property on="Test Slider" class="Slide (strict)"("Visible"=w260) -> ()  [unwired: 2 in, 2 out]
          }
          frame "Analog Out", "Motor", "PWM" {
            w266 = FALSE ("Visible")
            n145 = case shown="\"Analog Out\"" w265 {
              tunnel: [1.0 ("Value") -1.0 ("Value") 0.0 ("Value")] -> w264
              tunnel: [255.0 ("Value") 1.0 ("Value") 5.0 ("Value")] -> w263
              tunnel: [128.0 ("Value") 0.0 ("Value") 0.0 ("Value")] -> w262
              tunnel: [64.0 ("Value") 0.5 ("Value") 1.0 ("Value")] -> w261
              frame "PWM" {
              }
              frame "Motor", Default {
              }
              frame "Analog Out" {
              }
            }
            n146 = property on="Motor" class="Clust (strict)"("Visible"=TRUE) -> ()  [unwired: 2 in, 2 out]
            n147 = property on="Value" class="Slide (strict)"("Value"=w262, "Scale.Minimum"=w264, "Scale.Maximum"=w263, "Scale.Increment"=w261) -> ()  [unwired: 2 in, 2 out]
            n148 = property on="On/Off" class="Bool (strict)"("Visible"=w266) -> ()  [unwired: 2 in, 2 out]
            n149 = property on="Test Slider" class="Slide (strict)"("Visible"=w266) -> ()  [unwired: 2 in, 2 out]
            n150 = property on="Test Ring" class="Ring (strict)"("Visible"=w266) -> ()  [unwired: 2 in, 2 out]
            n151 = property on="Rev/Fwd" class="Clust (strict)"("Visible"=w266) -> ()  [unwired: 2 in, 2 out]
          }
          frame "Servo" {
            w282 = FALSE ("Visible")
            n152 = call <vilib>:"NT Read Number.vi"("Name"=w284) -> ("Numeric"=w283:dbl)  [unwired: 9 in, 1 out]
            n153 = property on="Test Slider" class="Slide (strict)"("Visible"=TRUE, "Scale.Maximum"=170.0 ("Scale.Range:Maximum")) -> ()  [unwired: 2 in, 2 out]
            n154 = local write "Test Slider"(w283) -> ()
            n155 = property on="Motor" class="Clust (strict)"("Visible"=w282) -> ()  [unwired: 2 in, 2 out]
            n156 = property on="Rev/Fwd" class="Clust (strict)"("Visible"=w282) -> ()  [unwired: 2 in, 2 out]
            n157 = property on="On/Off" class="Bool (strict)"("Visible"=w282) -> ()  [unwired: 2 in, 2 out]
            n158 = property on="Test Ring" class="Ring (strict)"("Visible"=w282) -> ()  [unwired: 2 in, 2 out]
          }
          frame "Relay", "Solenoid" {
            w285 = FALSE ("Visible")
            n159 = property on="Motor" class="Clust (strict)"("Visible"=w285) -> ()  [unwired: 2 in, 2 out]
            n160 = property on="Test Slider" class="Slide (strict)"("Visible"=w285) -> ()  [unwired: 2 in, 2 out]
            n161 = Search and Replace String(input string=w286, search string="/Value  **", replace string="/Direction") -> (result string=w292:string)  [unwired: 5 in, 3 out]
            n162 = property on="Test Ring" class="Ring (strict)"("Visible"=w285) -> ()  [unwired: 2 in, 2 out]
            n163 = call <vilib>:"NT Read String.vi"("Name"=w292) -> ("String"=w290:string)  [unwired: 9 in, 1 out]
            n164 = Equal?(x="Both directions", y=w290) -> (x = y?=w288:bool)
            n165 = Not(x=w288) -> (.not. x?=w289:bool)
            n166 = property on="Rev/Fwd" class="Clust (strict)"("Visible"=w288) -> ()  [unwired: 2 in, 2 out]
            n167 = property on="On/Off" class="Bool (strict)"("Visible"=w289, "Caption.Text"=w287) -> ()  [unwired: 2 in, 2 out]
          }
          frame "Compressor", "Digital Out" {
            w295 = FALSE ("Visible")
            # "Get direction and finish"
            n168 = property on="Motor" class="Clust (strict)"("Visible"=w295) -> ()  [unwired: 2 in, 2 out]
            n169 = property on="Test Slider" class="Slide (strict)"("Visible"=w295) -> ()  [unwired: 2 in, 2 out]
            n170 = property on="Test Ring" class="Ring (strict)"("Visible"=w295) -> ()  [unwired: 2 in, 2 out]
            n171 = property on="On/Off" class="Bool (strict)"("Visible"=TRUE, "Caption.Text"=w296) -> ()  [unwired: 2 in, 2 out]
            n172 = property on="Rev/Fwd" class="Clust (strict)"("Visible"=FALSE) -> ()  [unwired: 2 in, 2 out]
          }
          frame "Camera" {
            n173 = call <vilib>:"Get Last Path Segment.vi"("String in"=w303) -> ("String out"=w304:string)  [unwired: 10 in]
            n174 = property on="On/Off" class="Bool (strict)"("Visible"=FALSE) -> ()  [unwired: 2 in, 2 out]
            n175 = property on="Motor" class="Clust (strict)"("Visible"=FALSE) -> ()  [unwired: 2 in, 2 out]
            n176 = property on="Rev/Fwd" class="Clust (strict)"("Visible"=FALSE) -> ()  [unwired: 2 in, 2 out]
            n177 = case shown="\"White Balance  **\"" w304 {
              tunnel: w303 -> [w310 w319 w328 w337 w346 _ w352]
              tunnel: w302 -> [w308 w316 w325 w334 w343 _ _]
              frame "Size  **" {
                n178 = Index Array(array=w308) -> (element=w307:cluster{string[]})  [unwired: 1 in]
                n179 = call <vilib>:"NT Read String.vi"("Name"=w310) -> ("String"=w309:string)  [unwired: 9 in, 1 out]
                n180 = Unbundle(w307) -> (w305:string[])
                n181 = Match First String(2:w305, 3:w309) -> (0:w306:i32)  [unwired: 1 out]
                n182 = property on="Test Ring" class="Ring (strict)"("Value"=w306, "Strings []"=w305) -> ()  [unwired: 2 in, 2 out]
                n183 = property on="Test Ring" class="Ring (strict)"("Visible"=TRUE) -> ()  [unwired: 2 in, 2 out]
                n184 = property on="Test Slider" class="Slide (strict)"("Visible"=FALSE) -> ()  [unwired: 2 in, 2 out]
              }
              frame "White Balance  **" {
                n185 = Index Array(array=w316, index=1) -> (element=w317:cluster{string[]})
                n186 = call <vilib>:"NT Read String.vi"("Name"=w319) -> ("String"=w318:string)  [unwired: 9 in, 1 out]
                n187 = Unbundle(w317) -> (w314:string[])
                n188 = Match First String(2:w314, 3:w318) -> (0:w313:i32)  [unwired: 1 out]
                n189 = property on="Test Ring" class="Ring (strict)"("Value"=w313, "Strings []"=w314) -> ()  [unwired: 2 in, 2 out]
                n190 = property on="Test Ring" class="Ring (strict)"("Visible"=TRUE) -> ()  [unwired: 2 in, 2 out]
                n191 = property on="Test Slider" class="Slide (strict)"("Visible"=FALSE) -> ()  [unwired: 2 in, 2 out]
              }
              frame "Exposure  **" {
                n192 = Index Array(array=w325, index=2) -> (element=w326:cluster{string[]})
                n193 = call <vilib>:"NT Read String.vi"("Name"=w328) -> ("String"=w327:string)  [unwired: 9 in, 1 out]
                n194 = Unbundle(w326) -> (w322:string[])
                n195 = Match First String(2:w322, 3:w327) -> (0:w323:i32)  [unwired: 1 out]
                n196 = property on="Test Ring" class="Ring (strict)"("Value"=w323, "Strings []"=w322) -> ()  [unwired: 2 in, 2 out]
                n197 = property on="Test Ring" class="Ring (strict)"("Visible"=TRUE) -> ()  [unwired: 2 in, 2 out]
                n198 = property on="Test Slider" class="Slide (strict)"("Visible"=FALSE) -> ()  [unwired: 2 in, 2 out]
              }
              frame "Exposure Priority  **" {
                n199 = Index Array(array=w334, index=3) -> (element=w335:cluster{string[]})
                n200 = call <vilib>:"NT Read String.vi"("Name"=w337) -> ("String"=w336:string)  [unwired: 9 in, 1 out]
                n201 = Unbundle(w335) -> (w331:string[])
                n202 = Match First String(2:w331, 3:w336) -> (0:w332:i32)  [unwired: 1 out]
                n203 = property on="Test Ring" class="Ring (strict)"("Value"=w332, "Strings []"=w331) -> ()  [unwired: 2 in, 2 out]
                n204 = property on="Test Ring" class="Ring (strict)"("Visible"=TRUE) -> ()  [unwired: 2 in, 2 out]
                n205 = property on="Test Slider" class="Slide (strict)"("Visible"=FALSE) -> ()  [unwired: 2 in, 2 out]
              }
              frame "Color Enable  **" {
                n206 = Index Array(array=w343, index=4) -> (element=w344:cluster{string[]})
                n207 = call <vilib>:"NT Read String.vi"("Name"=w346) -> ("String"=w345:string)  [unwired: 9 in, 1 out]
                n208 = Unbundle(w344) -> (w340:string[])
                n209 = Match First String(2:w340, 3:w345) -> (0:w341:i32)  [unwired: 1 out]
                n210 = property on="Test Ring" class="Ring (strict)"("Value"=w341, "Strings []"=w340) -> ()  [unwired: 2 in, 2 out]
                n211 = property on="Test Ring" class="Ring (strict)"("Visible"=TRUE) -> ()  [unwired: 2 in, 2 out]
                n212 = property on="Test Slider" class="Slide (strict)"("Visible"=FALSE) -> ()  [unwired: 2 in, 2 out]
              }
              frame Default {
                n213 = property on="Test Ring" class="Ring (strict)"("Visible"=FALSE) -> ()  [unwired: 2 in, 2 out]
                n214 = property on="Test Slider" class="Slide (strict)"("Visible"=FALSE) -> ()  [unwired: 2 in, 2 out]
              }
              frame "Brightness  **", "Color Level  **", "Compression  **", "FPS  **", "Sharpness  **" {
                n215 = call <vilib>:"NT Read Number.vi"("Name"=w352) -> ("Numeric"=w351:dbl)  [unwired: 9 in, 1 out]
                n216 = local write "Test Slider"(w351) -> ()
                n217 = property on="Test Slider" class="Slide (strict)"("Visible"=TRUE, "Scale.Maximum"=100.0 ("Scale.Range:Maximum")) -> ()  [unwired: 2 in, 2 out]
                n218 = property on="Test Ring" class="Ring (strict)"("Visible"=FALSE) -> ()  [unwired: 2 in, 2 out]
              }
            }
          }
        }
        n219 = property on="Progress" class="Clust (strict)"("Visible"=FALSE) -> ()  [unwired: 2 in, 2 out]
      }
      event "Test Name": Mouse Enter {
        # "Populate the ring with the list of tests"
        n220 = event-data() -> ()  [unwired: 1 in, 1 out]
        n221 = call <vilib>:"NT Read String Array.vi"("Name"="TestMode/TestList") -> ("String Array"=w360:string[])  [unwired: 9 in, 1 out]
        n222 = Build Array (concatenate)("Select the test to run...", w360) -> (w359:string[])
        n223 = property on="Test Name" class="Ring (strict)"("Strings []"=w359) -> ()  [unwired: 2 in, 2 out]
      }
      event "Test Name": Value Change {
        w362 = FALSE ("Visible")
        # "Tell the robot the test name to run"
        n224 = event-data() -> ("NewVal"=w366:u16)  [unwired: 1 in]
        n225 = property on="Test Name" class="Ring (strict)"() -> ("Strings []"=w367:string[])  [unwired: 2 in, 2 out]
        n226 = local write "Progress"(T6 {"Test Progress"=0, "Test Progress Text"=""} ("Progress")) -> ()
        n227 = Index Array(array=w367, index=w366) -> (element=w365:string)
        n228 = call <vilib>:"NT Write String.vi"("String"=w365, "Name"="TestMode/TestName") -> ()  [unwired: 9 in, 1 out]
        n229 = property on="Progress" class="Clust (strict)"("Visible"=TRUE) -> ()  [unwired: 2 in, 2 out]
        n230 = property on="Motor" class="Clust (strict)"("Visible"=w362) -> ()  [unwired: 2 in, 2 out]
        n231 = property on="Test Slider" class="Slide (strict)"("Visible"=w362) -> ()  [unwired: 2 in, 2 out]
        n232 = property on="On/Off" class="Bool (strict)"("Visible"=w362) -> ()  [unwired: 2 in, 2 out]
        n233 = property on="Rev/Fwd" class="Clust (strict)"("Visible"=w362) -> ()  [unwired: 2 in, 2 out]
        n234 = property on="Test Ring" class="Ring (strict)"("Visible"=w362) -> ()  [unwired: 2 in, 2 out]
      }
      event "Select Auto": Mouse Enter {
        # "Populate the combo box with the list of autonomous options"
        n235 = event-data() -> ()  [unwired: 1 in, 1 out]
        n236 = call <vilib>:"NT Read String Array.vi"("Name"="Auto List") -> ("String Array"=w369:string[])  [unwired: 9 in, 1 out]
        n237 = property on="Select Auto" class="CmbBox"("Strings[]"=w369) -> ()  [unwired: 2 in, 2 out]
      }
      event "Select Auto": Value Change {
        # "User modified the Auto Selection. Write to NT variable so robot knows."
        n238 = event-data() -> ("NewVal"=w372:string)  [unwired: 1 in]
        n239 = call <vilib>:"NT Write String.vi"("String"=w372, "Name"="Auto Selector") -> ()  [unwired: 9 in, 1 out]
      }
      event "Command Selection": Value Change {
        # "Get the params and show in table"
        n240 = event-data() -> ("NewVal"=w378:i32)  [unwired: 1 in]
        n241 = property on="Command Selection" class="MCListbox (strict)"() -> ("ItemNames"=w376:string[][])  [unwired: 2 in, 2 out]
        n242 = call <vilib>:"WPI_DashboardUpdate Command Params.vi"("NewVal"=w378, "Commands"=w376, "Param Tbl"=w377) -> ()  [unwired: 8 in, 1 out]
      }
      event "Execute Command": Value Change {
        # "Started one, Unique ID holds\nresponse"
        n243 = event-data() -> ()  [unwired: 1 in, 1 out]
        n244 = property on="Command Selection" class="MCListbox (strict)"() -> ("ItemNames"=w389:string[][])  [unwired: 2 in, 2 out]
        n245 = Index Array(array=w389, index (row)="Command Selection", index (col)=0) -> (element=w387:string)
        n246 = call <vilib>:"Invoke Commands.vi"("Command Params"="Command Params", "Function Name"=w387) -> ("Params"=w383:u8, "Started"=w382:bool)  [unwired: 7 in, 1 out]
        n247 = Array Subset(array="Command Params", length (row)=w383) -> (w384:string[][])  [unwired: 3 in]
        n248 = Select(t="Executing" ("Cmd Status"), s=w382, f="" ("Cmd Status")) -> (s? t:f=→"Cmd Status":string)
      }
      event "Command Selection": Double Click {
        n249 = event-data() -> ("Row"=w397:i32)  [unwired: 1 in]
        n250 = property on="Command Selection" class="MCListbox (strict)"() -> ("ItemNames"=w400:string[][])  [unwired: 2 in, 2 out]
        n251 = local read "Command Params"() -> (w396:string[][])
        n252 = Index Array(array=w400, index (row)=w397, index (col)=0) -> (element=w398:string)
        n253 = call <vilib>:"Invoke Commands.vi"("Command Params"=w396, "Function Name"=w398) -> ("Params"=w395:u8, "Started"=w390:bool)  [unwired: 7 in, 1 out]
        n254 = Array Subset(array=w396, length (row)=w395) -> (w394:string[][])  [unwired: 3 in]
        n255 = Select(t="Executing" ("Cmd Status"), s=w390, f="" ("Cmd Status")) -> (s? t:f=w391:string)
        n256 = local write "Cmd Status"(w391) -> ()
      }
      event "CheckList": Double Click {
        # "Shift clears all"
        # "Update symbols on the listbox"
        n257 = event-data() -> ("PlatMods.Shift"=w402:bool, "Row"=w404:i32)  [unwired: 1 in]
        n258 = case shown="True" w402 {
          tunnel: w404 -> [w408 _]
          tunnel: 1 -> [w407 _]
          frame False {
            n259 = property on="CheckList" class="LstBox (strict)"() -> ("Item Symbols"=w406:i32[])  [unwired: 2 in, 2 out]
            n260 = Replace Array Subset(array=w406, new element=w407, index=w408) -> (w405:i32[])
            n261 = property on="CheckList" class="LstBox (strict)"("Item Symbols"=w405) -> ()  [unwired: 2 in, 2 out]
          }
          frame True {
            w409 = 0 ("Top Row")
            n262 = property on="CheckList" class="LstBox (strict)"() -> ("Number of Rows"=w411:u32)  [unwired: 2 in, 2 out]
            n263 = Initialize Array(0, w411) -> (w410:i32[])
            n264 = property on="CheckList" class="LstBox (strict)"("Top Row"=w409, "Value"=w409, "Item Symbols"=w410) -> ()  [unwired: 2 in, 2 out]
          }
        }
      }
      event "CheckList": Key Down {
        # "Update symbols on the listbox\nLeft and right keys check and uncheck"
        n265 = event-data() -> ("VKey"=w415:T22)  [unwired: 1 in]
        n266 = case shown="\"Left\", \"Right\"" w415 {
          selector: w415 -> [w420 _]
          tunnel: eventvkey."Left" ("VKey") -> [w418 _]
          frame "Left", "Right" {
            n267 = Equal?(x=w418, y=w420) -> (x = y?=w419:bool)
            n268 = Select(t=0, s=w419, f=1) -> (s? t:f=w421:i32)
            n269 = property on="CheckList" class="LstBox (strict)"() -> ("Item Symbols"=w424:i32[])  [unwired: 2 in, 2 out]
            n270 = Replace Array Subset(array=w424, new element=w421, index="CheckList") -> (w423:i32[])
            n271 = property on="CheckList" class="LstBox (strict)"("Item Symbols"=w423) -> ()  [unwired: 2 in, 2 out]
          }
          frame Default {
          }
        }
      }
      event "Motor.Enable": Value Change {
        # "When the test mode otor enable helper is set, update that\ntree row item's value"
        n272 = event-data() -> ("NewVal"=w430:bool)  [unwired: 1 in]
        n273 = Unbundle("Motor") -> ("Value"=w429:dbl)  [unwired: 1 out]
        n274 = Select(t=w429, s=w430, f=0.0) -> (s? t:f=w427:dbl)
        n275 = call <vilib>:"NT Write Number.vi"("Numeric"=w427, "Name"=w426) -> ()  [unwired: 9 in, 1 out]
      }
      event "Test Slider": Value Change {
        # "When the test mode slider helper is set, update that\ntree row item's value"
        n276 = event-data() -> ("NewVal"=w433:dbl)  [unwired: 1 in]
        n277 = call <vilib>:"NT Write Number.vi"("Numeric"=w433, "Name"=w434) -> ()  [unwired: 9 in, 1 out]
      }
      event "On/Off": Value Change {
        # "When the test mode on/off helper value is set, update that\ntree row item's value"
        n278 = event-data() -> ("NewVal"=w438:bool)  [unwired: 1 in]
        n279 = Boolean To (0,1)(Boolean=w438) -> (0, 1=w437:i16)
        n280 = call <vilib>:"NT Write Number.vi"("Numeric"=w437, "Name"=w436) -> ()  [unwired: 9 in, 1 out]
      }
      event "Rev/Fwd": Value Change {
        # "When the test mode helper value for relays is set, update that\ntree row item's value"
        n281 = event-data() -> ("NewVal.Forward"=w446:bool, "NewVal.Reverse"=w445:bool)  [unwired: 1 in]
        n282 = Boolean To (0,1)(Boolean=w446) -> (0, 1=w442:i16)
        n283 = Boolean To (0,1)(Boolean=w445) -> (0, 1=w444:i16)
        n284 = Negate(x=w444) -> (-x=w443:i16)
        n285 = Add(x=w442, y=w443) -> (x+y=w441:i16)
        n286 = call <vilib>:"NT Write Number.vi"("Numeric"=w441, "Name"=w440) -> ()  [unwired: 9 in, 1 out]
      }
      event "Test Ring": Value Change {
        # "When a test mode helper value is selected from the ring,\nset the tree item's variable to the string value"
        n287 = event-data() -> ("NewVal"=w450:u16)  [unwired: 1 in]
        n288 = property on="Test Ring" class="Ring (strict)"() -> ("Strings []"=w451:string[])  [unwired: 2 in, 2 out]
        n289 = Index Array(array=w451, index=w450) -> (element=w449:string)
        n290 = call <vilib>:"NT Write String.vi"("String"=w449, "Name"=w448) -> ()  [unwired: 9 in, 1 out]
      }
      event "Rec Mode": Value Change {
        # "Update globals for recording mode and path to read log from.\nClear when logging and let NetworkTables set path for vision to\nuse."
        n291 = event-data() -> ("NewVal"=w462:enum32{"Stop", "Record", "Playback"})  [unwired: 1 in]
        n292 = global write "WPI_DashboardLogging Global.vi" "Logging Filename"(path "") -> ()
        n293 = global write "WPI_DashboardLogging Global.vi" "Recording"(w462) -> ()
        n294 = case shown="\"Playback\"" w462 {
          tunnel: w461 -> [_ w464 w473]
          tunnel: [_ _ w472] -> w459
          tunnel: [_ _ w471] -> _
          tunnel: w457 -> [_ _ w469]
          tunnel: cluster{i32, i32} {-250, 170} -> [_ _ w468]
          tunnel: [_ _ T23 {"Image Size"=TRUE, "Image Type"=TRUE, "Pixel Value"=TRUE, "ROI Information"=TRUE, "Zoom Factor"=FALSE} ("Image Information Shown:All Elements")] -> w452
          tunnel: [_ _ TRUE ("Zoom Factor")] -> w453
          tunnel: w455 -> [_ _ w465]
          frame Default {
          }
          frame "Stop", "Record" {
            # "Place Window too"
            n295 = invoke class="VI" method="FP.Close"(reference=w464) -> (reference out=w463:refnum<vi>)  [unwired: 2 in, 2 out]
            n296 = invoke class="VI" method="Abort VI"(reference=w463) -> ()  [unwired: 2 in, 3 out]
          }
          frame "Playback" {
            n297 = call "Open Playback Panel.vi"("Offset"=w468, "DB VI Ref"=w469, "Playback in"=w473) -> ("Playback out"=w470:refnum<vi>)  [unwired: 8 in]
            n298 = register-events(w470, w465) -> (reference out=w472:refnum<event-registration>, error out=w471:errorcluster)  [unwired: 2 in]
          }
        }
        n299 = property on="Camera Image Right" class="ImageControl"("Image Information Shown"=w452, "Image Information Visible"=w453) -> ()  [unwired: 2 in, 2 out]
        n300 = property on="Camera Image" class="ImageControl"("Image Information Shown"=w452, "Image Information Visible"=w453) -> ()  [unwired: 2 in, 2 out]
        n301 = call <vilib>:"WPI_DashboardNT Log FieldName Cache.vi"("Operation"=enum16{"Lookup/Add", "Index", "Clear"}."Clear") -> ()  [unwired: 8 in, 3 out]
      }
      event Panel Close {
        w475 = enum32{"Stop", "Record", "Playback"}."Stop" ("Rec Mode")
        # "Playback window has been closed, abort"
        n302 = event-data() -> ()  [unwired: 1 in, 4 out]
        n303 = local write "Rec Mode"(w475) -> ()
        n304 = global write "WPI_DashboardLogging Global.vi" "Recording"(w475) -> ()
      }
      event Panel Close {
        # "Abort playback window and ourself"
        n305 = event-data() -> ()  [unwired: 1 in, 4 out]
        n306 = invoke class="VI" method="FP.Close"(reference=w479) -> (reference out=w478:refnum<vi>)  [unwired: 2 in, 2 out]
        n307 = invoke class="VI" method="Abort VI"(reference=w478) -> (error out=w477:errorcluster)  [unwired: 2 in, 2 out]
        n308 = invoke class="VI" method="Abort VI"(error in=w477) -> ()  [unwired: 2 in, 3 out]
      }
      event User Event {
        n309 = event-data() -> ("IDs"=w486:cluster{"RPC field ID":u16, "Unique ID":u16}, "String"=w485:string)  [unwired: 1 in]
        n310 = Bundle("IDs"=w486, "String"=w485) -> (w484:T9)  [unwired: 1 in]
        n311 = call <vilib>:"Retrieve RPC Response.vi"("RPC Response"=w484) -> ("Output"=w482:string[][])  [unwired: 10 in]
        n312 = Build Array (concatenate)(w480, w482) -> (w481:string[][])
        n313 = local write "Command Params"(w481) -> ()
        n314 = local write "Cmd Status"("" ("Cmd Status")) -> ()
      }
      event "Tree": Double Click {
        n315 = event-data() -> ("PlatMods"=w492:T26, "Tag"=w489:string)  [unwired: 1 in]
        n316 = Unbundle(w492) -> ("Shift"=w491:bool)  [unwired: 4 out]
        n317 = String Subset(string=w489, length (rest)=1 ("length (rest)")) -> (substring=w488:string)  [unwired: 1 in]
        n318 = Not(x=w491) -> (.not. x?=w490:bool)
        n319 = case shown="\"/\"" w488 {
          tunnel: w489 -> [_ w495]
          tunnel: w490 -> [_ w494]
          frame Default {
          }
          frame "/" {
            n320 = call <vilib>:"NT Update Persistence.vi"("Persistence"=w494, "Name"=w495) -> ()  [unwired: 9 in, 1 out]
          }
        }
      }
    }
  }
  n321 = while {
    tunnel: w65 -> [w497]
    i -> [w500]
    stop <- FALSE stop-if-true
    n322 = Wait (ms)(milliseconds to wait=u32 100) -> ()  [unwired: 1 out]
    n323 = case shown="\"Playback\"" "Rec Mode" {
      tunnel: w500 -> [_ _ w515]
      tunnel: [u32 2829099 ("Base Color") u32 11141120 ("Target Color") w504] -> w496
      frame "Stop", Default {
        # "Reset the color, extra updates don't cost much"
      }
      frame "Record" {
      }
      frame "Playback" {
        # "Playback"
        n324 = Quotient & Remainder(x=w515, y=u32 50 ("milliseconds to wait")) -> (x-y*floor(x/y)=w511:u32)  [unwired: 1 out]
        n325 = Divide(x=w511, y=u32 50 ("milliseconds to wait")) -> (x/y=w508:dbl)
        n326 = Multiply(x=6.283185307179586, y=w508) -> (x*y=w513:dbl)
        n327 = Sine(x=w513) -> (sin(x)=w512:dbl)
        n328 = Absolute Value(x=w512) -> (abs(x)=w505:dbl)
        n329 = call "Interpolate RGB Color.vi"("Proportion"=w505, "Target Color"=u32 30976, "Base Color"=u32 2829099) -> ("Result Color"=w504:u32)  [unwired: 8 in]
      }
    }
    n330 = property class="Pane"(reference=w497, "PaneColor"=w496) -> ()  [unwired: 1 in, 2 out]
  }
  n331 = local write "Dashboard Tab"(T2."Drive" ("Dashboard Tab")) -> ()
  n332 = property on="On/Off" class="Bool (strict)"("Visible"=w36) -> ()  [unwired: 2 in, 2 out]
  n333 = property on="Motor" class="Clust (strict)"("Visible"=w36) -> ()  [unwired: 2 in, 2 out]
  n334 = property on="Progress" class="Clust (strict)"("Visible"=w36) -> ()  [unwired: 2 in, 2 out]
  n335 = property on="Test Ring" class="Ring (strict)"("Visible"=w36) -> ()  [unwired: 2 in, 2 out]
  n336 = property on="Rev/Fwd" class="Clust (strict)"("Visible"=w36) -> ()  [unwired: 2 in, 2 out]
  n337 = local write "Command Selection"(u16 0 ("milliseconds to wait")) -> ()
  n338 = while {
    tunnel: u16 1741 ("timeout ms (25000)") -> [w517]
    stop <- FALSE stop-if-true
    n339 = TCP Create Listener(10:w517) -> (0:w516:errorcluster, 3:w518:refnum<k5>)  [unwired: 4 in, 1 out]
    n340 = case shown="No Error" w516 {
      selector: w516 -> [w520 _]
      tunnel: w518 -> [w521 _]
      frame No Error {
        n341 = while {
          tunnel: w521 -> [w524]
          tunnel: w520 -> [w523]
          stop <- FALSE stop-if-true
          n342 = TCP Wait On Listener(8:w523, 11:w524) -> (0:w525:errorcluster, 4:w526:refnum<k5>)  [unwired: 2 in, 3 out]
          n343 = local write "TCP"(w526) -> ()
          n344 = case shown="No Error" w525 {
            frame No Error {
            }
            frame Error {
              n345 = Wait (ms)(milliseconds to wait=u32 1000) -> ()  [unwired: 1 out]
            }
          }
        }
      }
      frame Error {
        n346 = Wait (ms)(milliseconds to wait=u32 1000) -> ()  [unwired: 1 out]
      }
    }
  }
  n347 = local write "Command Params"(string[][] [] ("Command Params")) -> ()
  n348 = global write "WPI_DashboardLogging Global.vi" "Recording"(w59) -> ()
  n349 = local write "Rec Mode"(w59) -> ()
  n350 = call <vilib>:"NT Write String.vi"("String"="Select Auto", "Name"="Auto Selector") -> ()  [unwired: 9 in, 1 out]
